vi "Q5_Tranformation.vi"(7 "Input Bit":dbl, 8 "Is Positive":enum16{"False", "True"}(ring), 9 "Q Factor":dbl, 10 "Coefficient":dbl, 11 "DLS ERD Data":dbl) -> (3 "Result Q5 Tranformation":dbl)   [LabVIEW 2016, in "TL27.lvlib"]
uses:
  Projects/TL27.lvlib
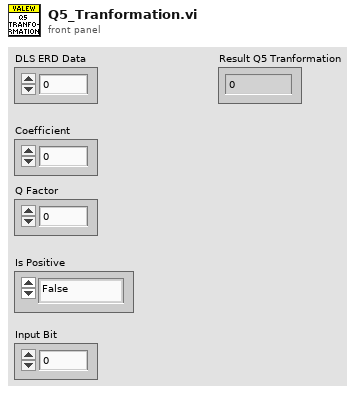
[diagram p1: front panel]
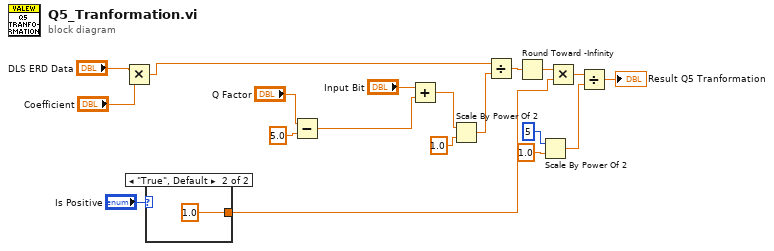
[diagram p0: block diagram]
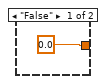
[diagram p2: hidden frame]
diagram:
  n1 = Multiply(x="DLS ERD Data", y="Coefficient") -> (x*y=w10:dbl)
  n2 = case shown="\"True\", Default" "Is Positive" {
    tunnel: [0.0 1.0] -> w12
    frame "False" {
    }
    frame "True", Default {
    }
  }
  n3 = Subtract(x="Q Factor", y=5.0) -> (x-y=w3:dbl)
  n4 = Add(x="Input Bit", y=w3) -> (x+y=w2:dbl)
  n5 = Scale By Power Of 2(n=w2, x=1.0) -> (x*2^n=w11:dbl)
  n6 = Divide(x=w10, y=w11) -> (x/y=w17:dbl)
  n7 = Round Toward -Infinity(1:w17) -> (0:w18:dbl)
  n8 = Scale By Power Of 2(n=i16 5, x=1.0) -> (x*2^n=w15:dbl)
  n9 = Multiply(x=w18, y=w12) -> (x*y=w19:dbl)
  n10 = Divide(x=w19, y=w15) -> (x/y=→"Result Q5 Tranformation":dbl)
